vi "Get Service Settings - PVM.vi"(8 "error in (no error)":errorcluster) -> (0 "error out":errorcluster, 3 "service settings":T1)   [LabVIEW 2021, in "AudioGenUtility.lvlib"]
uses:
  controls/service settings.ctl
  AudioGenUtility.lvlib
  <vilib>/addons/PointValueMap/PointValueMap.lvlib
  <vilib>/addons/PointValueMap/subVIs/Point_Write_variant.vi
  <vilib>/addons/PointValueMap/subVIs/Point_Read_variant.vi
  controls/AudioGenTypeDefs.lvlib
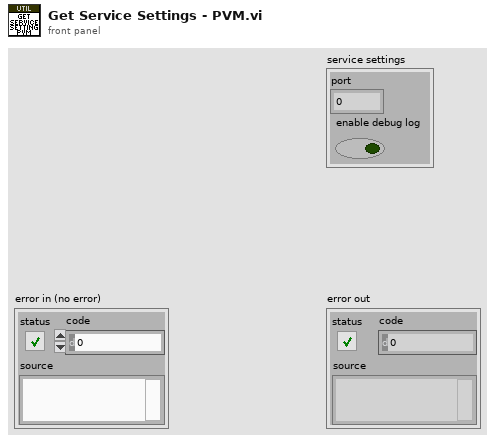
[diagram p1: front panel]
types:
  T1 = typedef "AudioGenTypeDefs.lvlib/service settings.ctl" = cluster{"port":u32, "enable debug log":bool}
  T2 = typedef "PointValueMap.lvlib/PointMap.ctl" = refnum<data-value>
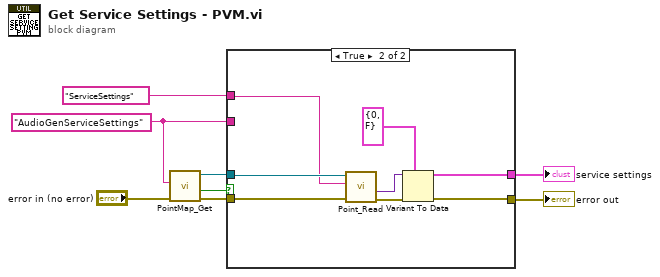
[diagram p0: block diagram]
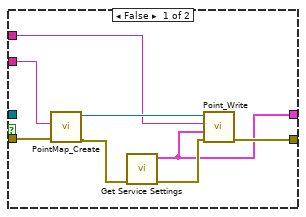
[diagram p2: hidden frame]
diagram:
  w4 = "AudioGenServiceSettings" ("process name")
  n1 = call <vilib>:"PointMap_Get.vi"("error in (no error)"="error in (no error)", "Name"=w4) -> ("error out"=w7:errorcluster, "Found?"=w8:bool, "Map Out"=w6:T2)  [unwired: 7 in]
  n2 = case shown="True" w8 {
    tunnel: w7 -> [w16 w24]
    tunnel: [w11 w17] -> w2
    tunnel: w6 -> [_ w23]
    tunnel: w4 -> [w15 _]
    tunnel: [w10 w18] -> w3
    tunnel: "ServiceSettings" ("Tag") -> [w9 w22]
    frame False {
      n3 = call <vilib>:"PointMap_Create.vi"("error in (no error)"=w16, "Name"=w15) -> ("error out"=w13:errorcluster, "Map Out"=w14:T2)  [unwired: 8 in]
      n4 = call "Get Service Settings.vi"("error in (no error)"=w13) -> ("error out"=w12:errorcluster, "service settings"=w10:T1)  [unwired: 9 in]
      n5 = call-poly <vilib>:"Point_Write.vi"("Error In"=w12, "Value"=w10, "Tag"=w9, "Map"=w14) -> ("Error Out"=w11:errorcluster)  [unwired: 6 in, 1 out]
    }
    frame True {
      n6 = call-poly <vilib>:"Point_Read.vi"("Error In"=w24, "Tag"=w22, "Map"=w23) -> ("Error Out"=w21:errorcluster, "Value"=w20:variant)  [unwired: 3 in, 4 out]
      n7 = Variant To Data(error in=w21, type=T1 {"port"=0, "enable debug log"=FALSE} ("service settings"), Variant=w20) -> (data=w18:T1, error out=w17:errorcluster)
    }
  }
  "error out" <- w2
  "service settings" <- w3
